vi "Get Bookmark VI Actions.vi"(8 "error in (no error)":errorcluster {"code" format="Error %.0f"}, 10 "Term":string, 11 "VIDoc Printer In":refnum<class "VIDoc Printer.lvclass">) -> (0 "error out":errorcluster {"code" format="Error %.0f"}, 2 "Bookmark VI Actions":T1[](array[typedef]), 3 "VIDoc Printer Out":refnum<class "VIDoc Printer.lvclass">)   [LabVIEW 2023, in "VIDoc Printer.lvlib" / "VIDoc Printer.lvclass"]
uses:
  VIDoc Printer.lvclass
  Controls/Process VI Enum.ctl
  VIDoc Printer.lvclass/VIDoc Printer.ctl
  Get VI Settings - Memory.vi
  Get VI Settings - By Folder.vi
  Get VI Settings - By Tree.vi
  Get VI Settings - By List.vi
  Get VI Settings - List Detail Level.vi
  Get VI Settings - Methods.vi
  Get VI Settings - Methods Detail Level.vi
  Get VI Settings - Method Options - Front Panels.vi
  Get VI Settings - Method Options - Options.vi
  Get VI Settings - Method Options - Controls.vi
  Get VI Settings - Controls Detail Level.vi
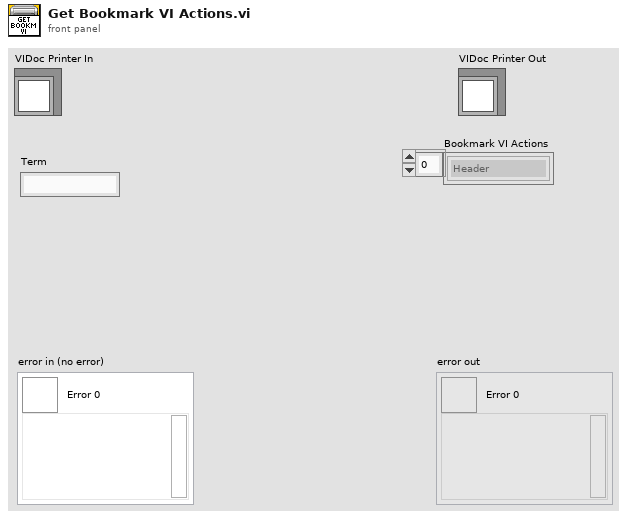
[diagram p1: front panel]
types:
  T1 = typedef "VIDoc Printer.lvlib/VIDoc Printer.lvclass/Process VI Enum.ctl" = enum16{"Header", "Memory", "By Folder", "By Tree", "By List", "Method Details", "FP"}
  T2 = typedef "VIDoc Printer.lvlib/Printer Settings.lvclass/VI Settings.ctl" = cluster{"Memory":bool, "By Folder":bool, "By Tree":bool, "By List":bool, "Methods":bool, "Method Options":cluster{"Front Panels":bool, "Options":bool, "Controls":bool}, "List Detail Level":T3, "Methods Detail Level":T3, "Controls Detail Level":T3}
  T3 = typedef "VIDoc Printer.lvlib/Printer Settings.lvclass/Detail Level Enum.ctl" = enum16{"None", "Minimal", "Standard", "Full"}
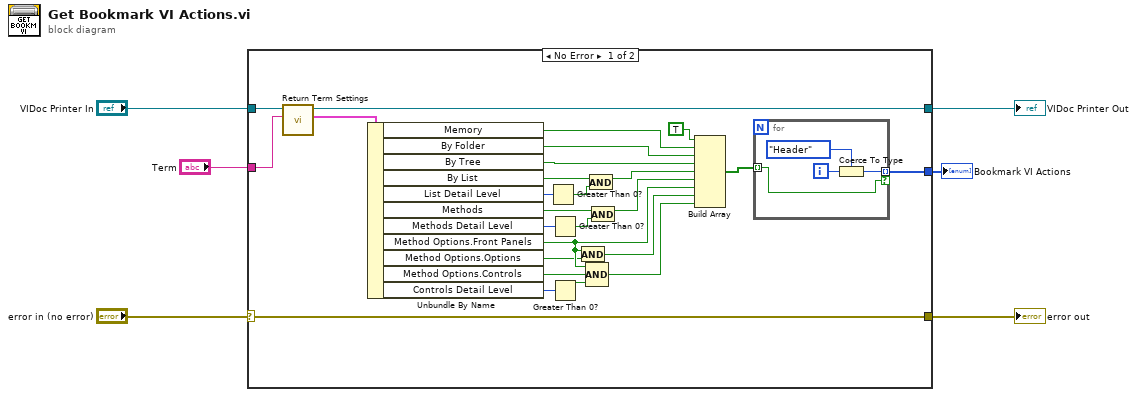
[diagram p0: block diagram]
diagram:
  n1 = case shown="No Error" "error in (no error)" {
    selector: "error in (no error)" -> [w32 w38]
    tunnel: [w32 w38] -> w5
    tunnel: [w7 w37] -> w3
    tunnel: "VIDoc Printer In" -> [w21 w37]
    tunnel: [w29 _] -> w2
    tunnel: "Term" -> [w20 _]
    frame No Error {
      n2 = call "Return Term Settings.vi"("Term"=w20, "Printer in"=w21) -> ("Term Settings"=w19:T2, "Printer out"=w7:refnum<class "VIDoc Printer.lvclass">)  [unwired: 6 in, 2 out]
      n3 = Unbundle By Name(w19) -> ("Memory"=w18:bool, "By Folder"=w17:bool, "By Tree"=w16:bool, "By List"=w15:bool, "List Detail Level"=w14:T3, "Methods"=w13:bool, "Methods Detail Level"=w12:T3, "Method Options.Front Panels"=w11:bool, "Method Options.Options"=w10:bool, "Method Options.Controls"=w9:bool, "Controls Detail Level"=w8:T3)
      n4 = Greater Than 0?(x=w14) -> (x > 0?=w27:bool)
      n5 = Greater Than 0?(x=w12) -> (x > 0?=w25:bool)
      n6 = Greater Than 0?(x=w8) -> (x > 0?=w23:bool)
      n7 = And(x=w11, y=w10) -> (x .and. y?=w24:bool)
      n8 = And(x=w15, y=w27) -> (x .and. y?=w28:bool)
      n9 = Compound Arithmetic op=AND(w11, w9, w23) -> (w22:bool)
      n10 = And(x=w13, y=w25) -> (x .and. y?=w26:bool)
      n11 = Build Array(TRUE ("element"), w18, w17, w16, w28, w26, w11, w24, w22) -> (w30:bool[])
      n12 = for {
        tunnel: w30 -> [w33] mode=indexing
        tunnel: [w34] -> w29 mode=indexing if=w33
        i -> [w35]
        n13 = Coerce To Type(0:w35, 1:Process_VI_Enum."Header") -> (2:w34:T1)
      }
    }
    frame Error {
    }
  }
  "error out" <- w5
  "VIDoc Printer Out" <- w3
  "Bookmark VI Actions" <- w2
